vi "helper.vi"() -> ()   [LabVIEW 2021]
panel:
  in  "Array":dbl[](array[numeric])
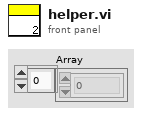
[diagram p1: front panel]
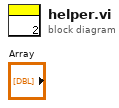
[diagram p0: block diagram]
diagram:
